vi "Poll Sample Push Control.vi"(8 "error in (no error)":errorcluster, 11 "cRIO-CO2 in":refnum<class "cRIO-CO2.lvclass">) -> (0 "error out":errorcluster, 3 "cRIO-CO2 out":refnum<class "cRIO-CO2.lvclass">)   [LabVIEW 2015, in "cRIO-Carbondioxide.lvlib" / "cRIO-CO2.lvlib" / "cRIO-CO2.lvclass"]
uses:
  cRIO-CO2.lvclass
  Controls/Sample Push Control Enumerator.ctl
  cRIO-CO2.lvclass/cRIO-CO2.ctl
  <vilib>/ActorFramework/Message Enqueuer/Message Enqueuer.lvclass/Message Enqueuer.ctl
  cRIO-CO2 Messages/Sample Push Reset to Idle Msg/Sample Push Reset to Idle Msg.lvclass/Sample Push Reset to Idle Msg.ctl
  <vilib>/ActorFramework/Message Enqueuer/Enqueue.vi
  <vilib>/ActorFramework/Message Priority Queue/Priority Enqueue.vi
  cRIO-CO2 Messages/Sample Push go for Push State Msg/Sample Push go for Push State Msg.lvclass
  cRIO-CO2 Messages/Sample Push go for Stash State Msg/Sample Push go for Stash State Msg.lvclass
  cRIO-CO2 Messages/Abort Sample Push Msg/Sample Push Abort Msg.lvclass
  cRIO-CO2 Messages/Sample Push Reset to Idle Msg/Sample Push Reset to Idle Msg.lvclass
panel:
  out "error IO":errorcluster
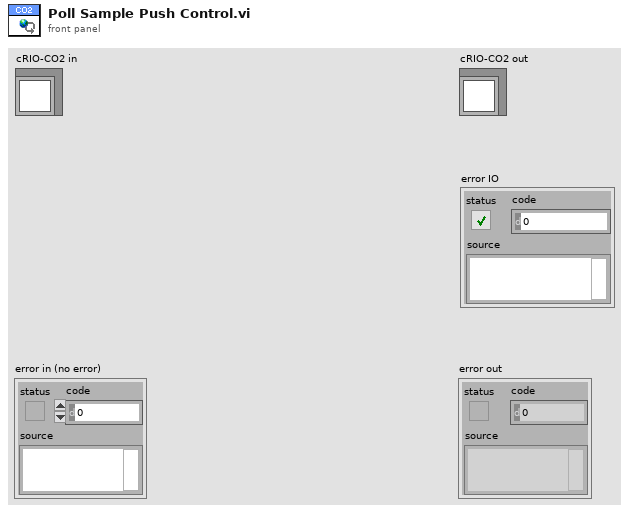
[diagram p1: front panel]
types:
  T1 = typedef "Sample Push Control Enumerator.ctl" = enum16{"Acknowledged", "Push", "Stash", "Abort", "Reset to Idle"}
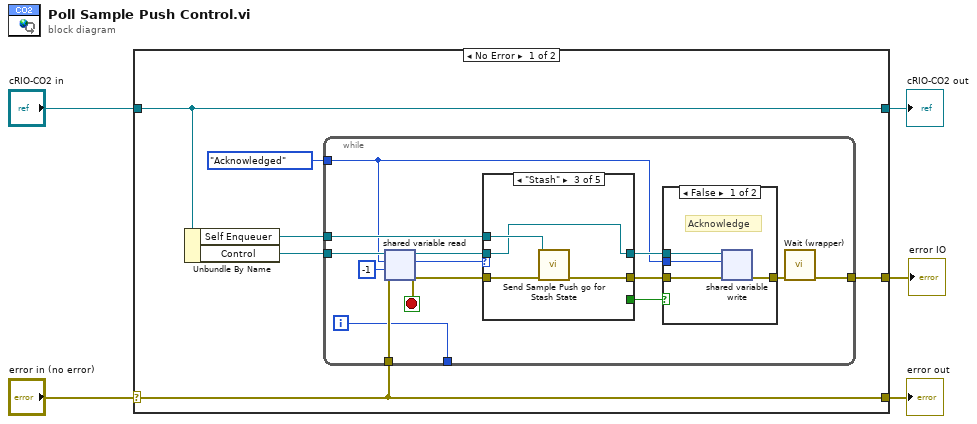
[diagram p0: block diagram]
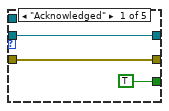
[diagram p3: hidden frame]
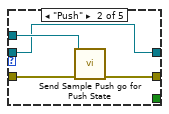
[diagram p4: hidden frame]
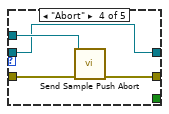
[diagram p5: hidden frame]
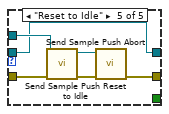
[diagram p6: hidden frame]
diagram:
  n1 = case shown="No Error" "error in (no error)" {
    selector: "error in (no error)" -> [w10 w53]
    tunnel: [w10 w53] -> w4
    tunnel: [w9 w52] -> w2
    tunnel: "cRIO-CO2 in" -> [w9 w52]
    tunnel: [w6 _] -> w1
    frame No Error {
      n2 = Unbundle By Name(w9) -> ("Self Enqueuer"=w7:refnum<class "Message Enqueuer.lvclass">, "Control"=w11:refnum<k21>)
      n3 = while {
        tunnel: w11 -> [w24]
        tunnel: w10 -> [w23]
        tunnel: Sample_Push_Control_Enumerator."Acknowledged" ("Sample Transfer Control") -> [w16]
        tunnel: [w14] -> w6
        tunnel: w7 -> [w17]
        tunnel: [w13] -> _
        i -> [w13]
        stop <- w21 stop-if-true
        n4 = shared-variable-read(w24, w23, w16, -1 ("timeout ms")) -> (w20:refnum<k21>, w21:errorcluster, w22:T1)  [unwired: 2 out]
        n5 = case shown="\"Stash\"" w22 {
          tunnel: w21 -> [w33 w37 w41 w45 w51]
          tunnel: [w33 w36 w39 w44 w46] -> w19
          tunnel: w20 -> [w32 w34 w38 w42 w47]
          tunnel: [w32 w34 w38 w42 w47] -> w18
          tunnel: w17 -> [_ w35 w40 w43 w50]
          tunnel: [TRUE _ _ _ _] -> w12
          frame "Acknowledged" {
          }
          frame "Push" {
            n6 = call "Send Sample Push go for Push State.vi"("error in (no error)"=w37, "Message Enqueuer"=w35) -> ("error out"=w36:errorcluster)  [unwired: 8 in, 1 out]
          }
          frame "Stash" {
            n7 = call "Send Sample Push go for Stash State.vi"("error in (no error)"=w41, "Message Enqueuer"=w40) -> ("error out"=w39:errorcluster)  [unwired: 8 in, 1 out]
          }
          frame "Abort" {
            n8 = call "Send Sample Push Abort.vi"("error in (no error)"=w45, "Message Enqueuer"=w43) -> ("error out"=w44:errorcluster)  [unwired: 8 in, 1 out]
          }
          frame "Reset to Idle" {
            n9 = call "Send Sample Push Abort.vi"("error in (no error)"=w51, "Message Enqueuer"=w50) -> ("error out"=w49:errorcluster, "Message Enqueuer out"=w48:refnum<class "Message Enqueuer.lvclass">)  [unwired: 8 in]
            n10 = call "Send Sample Push Reset to Idle.vi"("error in (no error)"=w49, "Message Enqueuer"=w48) -> ("error out"=w46:errorcluster)  [unwired: 8 in, 1 out]
          }
        }
        n11 = case shown="False" w12 {
          tunnel: w19 -> [w29 w30]
          tunnel: w18 -> [w28 _]
          tunnel: w16 -> [w27 _]
          tunnel: [w26 w30] -> w15
          frame False {
            # "Acknowledge"
            n12 = shared-variable-write(w28, w29, w27) -> (w26:errorcluster)  [unwired: 1 out]
          }
          frame True {
          }
        }
        n13 = call "Wait (wrapper).vi"("error in (no error)"=w15) -> ("error out"=w14:errorcluster)  [unwired: 10 in]
      }
    }
    frame Error {
    }
  }
  "error out" <- w4
  "cRIO-CO2 out" <- w2
  "error IO" <- w1
